vi "Global Release.vi"(8 "error in (no error)":errorcluster, 11 "Global":refnum<k1>) -> (0 "error out":errorcluster)   [LabVIEW 2022 SP3, in "Shared.lvlib"]
uses:
  Shared.lvlib
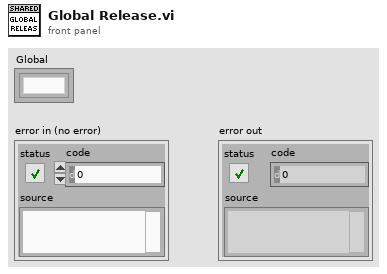
[diagram p1: front panel]
types:
  T1 = cluster{"Global":cluster{"ID":i32, "Name":string, "Parent":i32, "Queue":refnum<queue>, "Ini Path":path, "Ini Section":string, "VI Name":string, "VI Path":path, "VI Refnum":refnum<vi>, "Group":string}[]}[]
  T2 = cluster{"Global":cluster{"ID":i32, "Name":string, "Parent":i32, "Queue":refnum<queue>, "Ini Path":path, "Ini Section":string, "VI Name":string, "VI Path":path, "VI Refnum":refnum<vi>, "Group":string}[]}
  T3 = cluster{"ID":i32, "Name":string, "Parent":i32, "Queue":refnum<queue>, "Ini Path":path, "Ini Section":string, "VI Name":string, "VI Path":path, "VI Refnum":refnum<vi>, "Group":string}[]
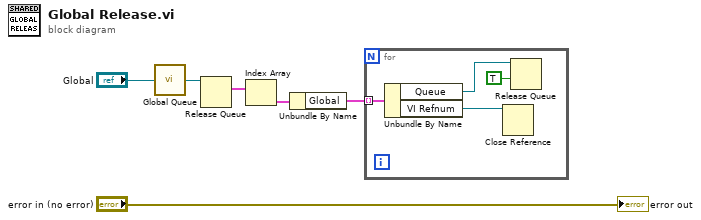
[diagram p0: block diagram]
diagram:
  n1 = call "Global Queue.vi"("Global in"="Global") -> ("Global"=w5:refnum<queue>)
  n2 = Release Queue(queue=w5) -> (remaining elements=w4:T1)  [unwired: 2 in, 2 out]
  n3 = Index Array(array=w4) -> (element=w3:T2)  [unwired: 1 in]
  n4 = Unbundle By Name(w3) -> ("Global"=w2:T3)
  n5 = for {
    tunnel: w2 -> [w10] mode=indexing
    n6 = Unbundle By Name(w10) -> ("Queue"=w9:refnum<queue>, "VI Refnum"=w8:refnum<vi>)
    n7 = Close Reference(reference=w8) -> ()  [unwired: 1 in, 1 out]
    n8 = Release Queue(queue=w9, force destroy? (F)=TRUE) -> ()  [unwired: 1 in, 3 out]
  }
  "error out" <- "error in (no error)"
